vi "Find Control in Cluster.vi"(8 "error in (no error)":errorcluster, 10 "control label":string, 11 "cluster reference in":refnum<vi>) -> (0 "error out":errorcluster, 2 "control reference":refnum<vi>, 3 "cluster reference out":refnum<vi>)   [LabVIEW 2015, in "PL Utility.lvlib"]
doc: "Finds control with a specified <b>control label</b> in the cluster specified by <b>cluster reference</b> and returns <b>control reference</b>."
uses:
  PL Utility.lvlib
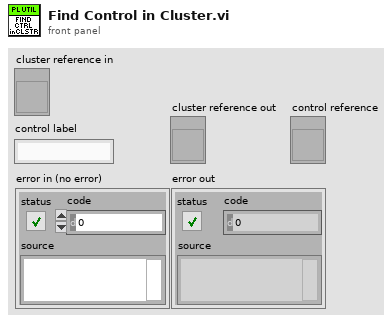
[diagram p1: front panel]
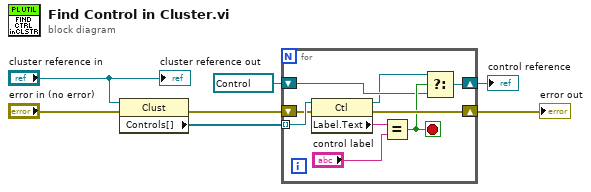
[diagram p0: block diagram]
diagram:
  n1 = property class="Clust"(reference="cluster reference in", error in="error in (no error)") -> (error out=w2:errorcluster, "Controls[]"=w1:refnum<vi>[])  [unwired: 1 out]
  n2 = for {
    tunnel: w1 -> [w16] mode=indexing
    shift-right: [w14] -> w6
    shift-left: w2 -> [w15]
    shift-right: [w10] -> w7
    shift-left: refnum<vi> refnum ("reference out") -> [w11]
    stop <- w12 stop-if-true
    n3 = property class="Ctl"(reference=w16, error in=w15) -> (reference out=w8:refnum<vi>, error out=w14:errorcluster, "Label.Text"=w13:string)
    n4 = Equal?(x=w13, y="control label") -> (x = y?=w12:bool)
    n5 = Select(t=w8, s=w12, f=w11) -> (s? t:f=w10:refnum<vi>)
  }
  "error out" <- w6
  "control reference" <- w7
  "cluster reference out" <- "cluster reference in"
